vi "Update Settings.vi"(7 "Multicolumn Listbox Ref In":refnum<vi>, 8 "Error In":errorcluster, 11 "eHS Matrix Generation Session Ref In":refnum<data-value>) -> (0 "Error Out":errorcluster, 3 "eHS Matrix Generation Session Ref Out":refnum<data-value>)   [LabVIEW 2017]
uses:
  <vilib>/OPAL-RT/eHS Toolkit/eHS Matrix Generation/_Controls/eHS Core Index.ctl
  <vilib>/OPAL-RT/eHS Toolkit/eHS Matrix Generation/_Controls/eHS Matrix Generation Session.ctl
  <vilib>/OPAL-RT/eHS Toolkit/eHS Matrix Generation/_Controls/eHS Target Information.ctl
  <vilib>/OPAL-RT/eHS Toolkit/eHS Matrix Generation/_Controls/eHS Matrix Generation Parameters.ctl
  <vilib>/OPAL-RT/eHS Toolkit/eHS Matrix Generation/_Controls/eHS Circuit Analysis Data.ctl
  <vilib>/OPAL-RT/eHS Toolkit/eHS Matrix Generation/_Controls/eHS Core Settings.ctl
  <vilib>/OPAL-RT/eHS Toolkit/eHS Matrix Generation/_Controls/eHS Form Factor.ctl
  <vilib>/OPAL-RT/eHS Toolkit/eHS Matrix Generation/_Controls/eHS Model Information.ctl
  Update Settings States.ctl
  UI Refs.ctl
  ListBox/ListBox Action.ctl
  <vilib>/OPAL-RT/eHS Toolkit/eHS Matrix Generation/eHS Matrix Generation.lvlib
panel:
  out "Support Scenarios?":bool
  in  "Gs Settings":cluster{"SW#":i32, "Gs":sgl}[](array[cluster]) {"SW#" format="%02d"}
  in  "eHS Form Factor":T1=enum."eHSx64"
  out "Desired Ts (s)":string
  out "Cur eHS Form Factor":string
  out "eHS Core Index":string
  out "Model Name":string
  in  "Change Core":bool
  in  "Get Settings":bool
  in  "Update?":bool
  in  "Desired Gs":dbl
  out "Number of Switches":string
  in  "Same Gs for all Switches?":bool
  in  "Desired Ts (s)":dbl
  in  "Done":bool
  out "Minimum Achievable Ts (s)":string
  out "Display":string
  in  "Choose eHS Core Index":T2
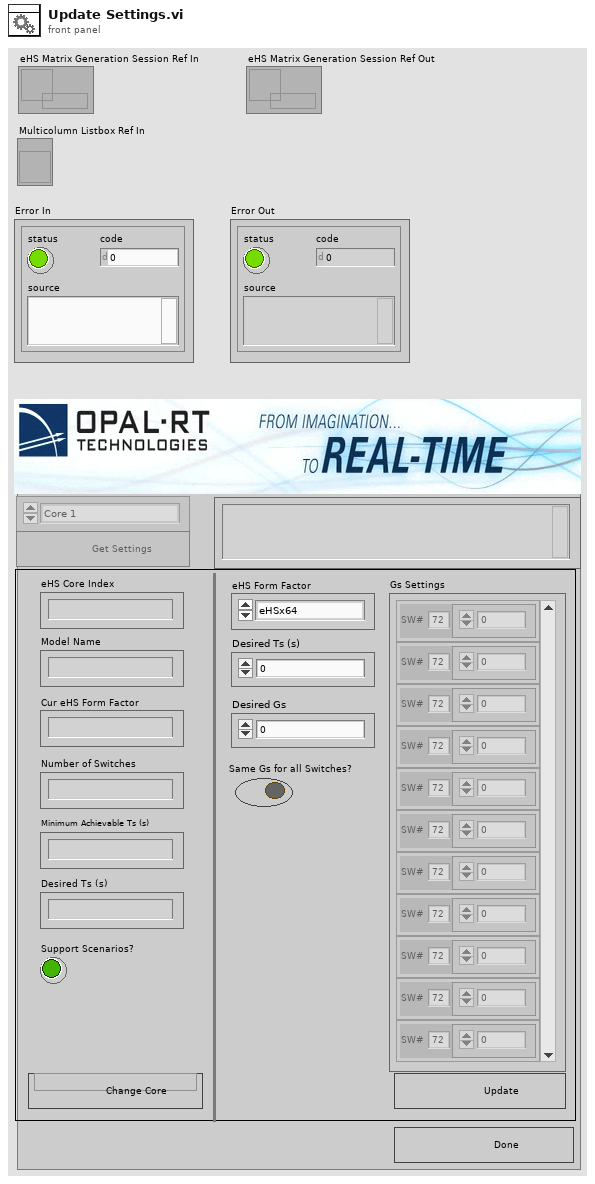
[diagram p1: front panel]
types:
  T1 = typedef "OPAL-RT eHS.lvlib/eHS Matrix Generation.lvlib/eHS Form Factor.ctl" = enum16{"eHSx16", "eHSx32", "eHSx64"}
  T2 = typedef "OPAL-RT eHS.lvlib/eHS Matrix Generation.lvlib/eHS Core Index.ctl" = enum16{"Core 1", "Core 2", "Core 3", "Core 4", "Core 5", "Core 6", "Core 7", "Core 8", "Core 9", "Core 10"}
  T3 = typedef "Update Settings States.ctl" = enum16{"Init", "Get Settings", "Update Settings", "Change Core", "Event Handler"}
  T4 = typedef "UI Refs.ctl" = cluster{"Choose Core":refnum<vi>, "Get Settings":refnum<vi>, "Change Core":refnum<vi>, "Form Factor":refnum<vi>, "Desired Ts":refnum<vi>, "Desired Gs":refnum<vi>, "Same Gs All":refnum<vi>, "Gs Settings":refnum<vi>, "Update":refnum<vi>}
  T5 = enum8{"Enabled", "Disabled", "Disabled and Grayed Out"}
  T6 = typedef "ListBox Action.ctl" = enum16{"Add", "Overwrite"}
  T7 = typedef "OPAL-RT eHS.lvlib/eHS Matrix Generation.lvlib/eHS Circuit Analysis Data.ctl" = cluster{"Number of Switches":string, "Desired Ts":string, "Gs":dbl[], "Min Ts":string}
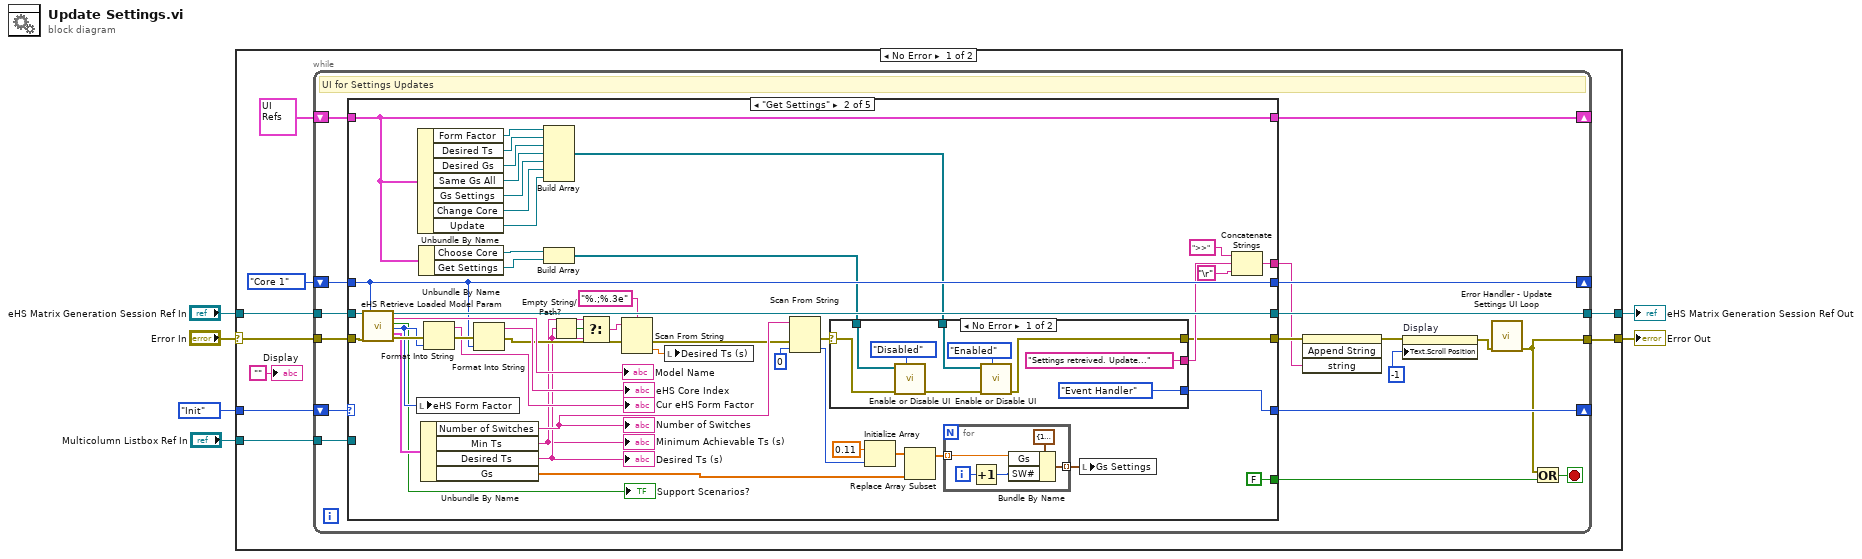
[diagram p0: block diagram]
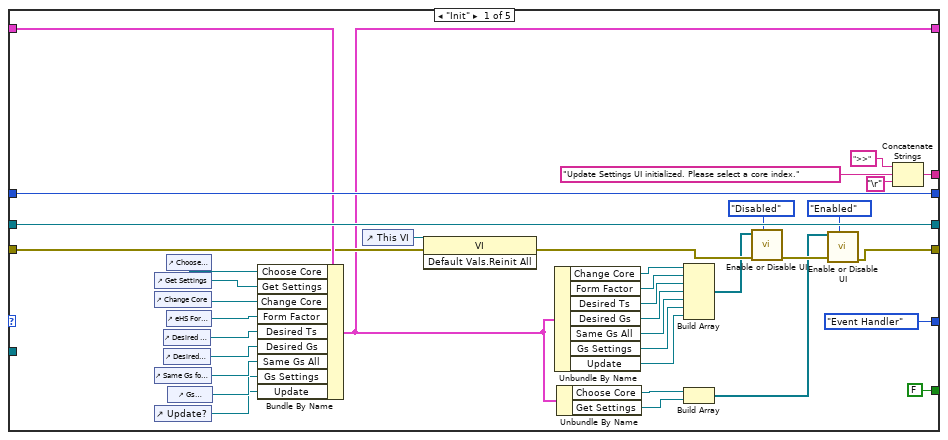
[diagram p2: hidden frame]
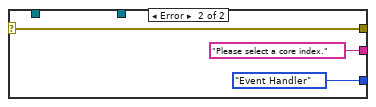
[diagram p3: hidden frame]
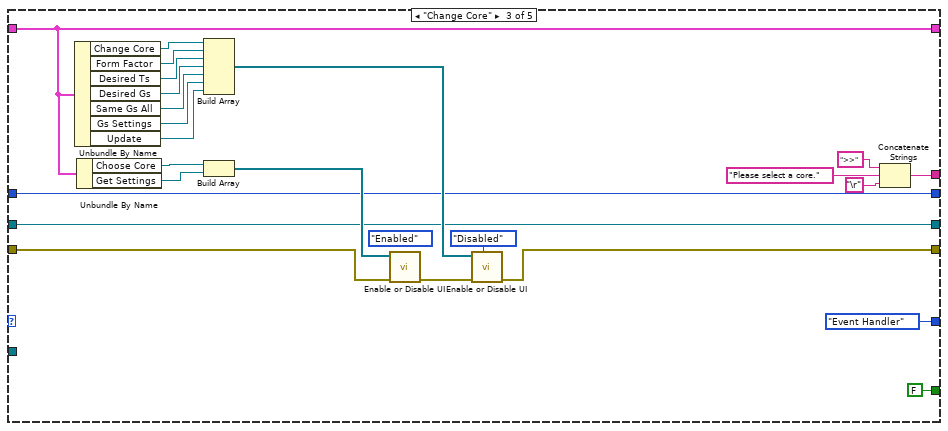
[diagram p4: hidden frame]
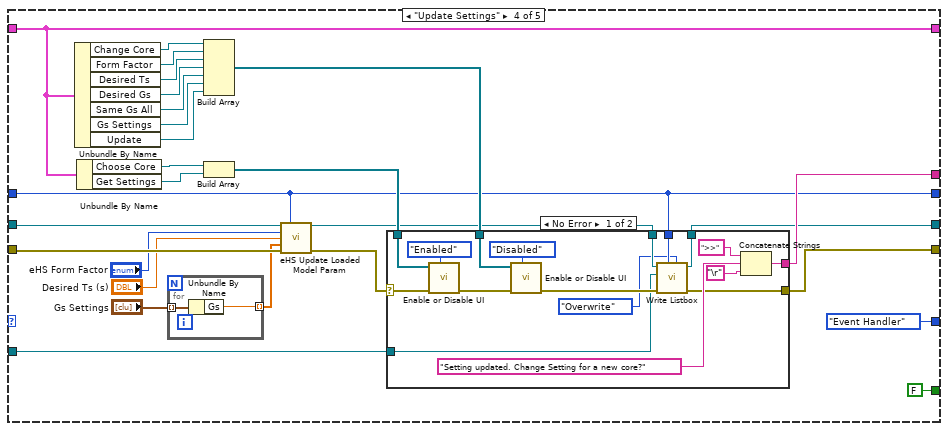
[diagram p5: hidden frame]
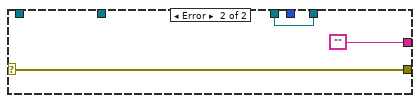
[diagram p6: hidden frame]
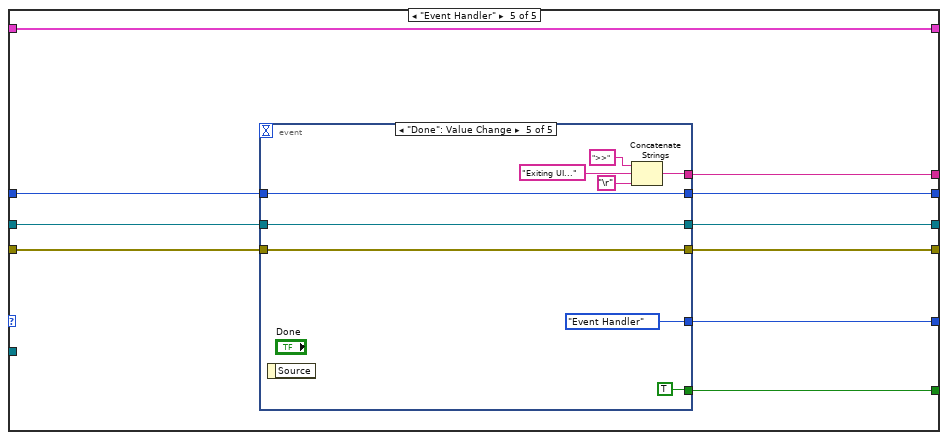
[diagram p7: hidden frame]
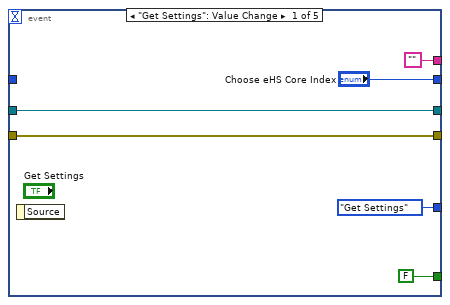
[diagram p8: hidden frame]
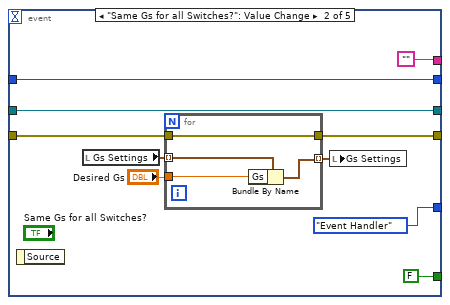
[diagram p9: hidden frame]
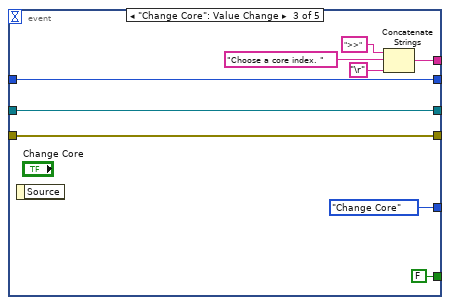
[diagram p10: hidden frame]
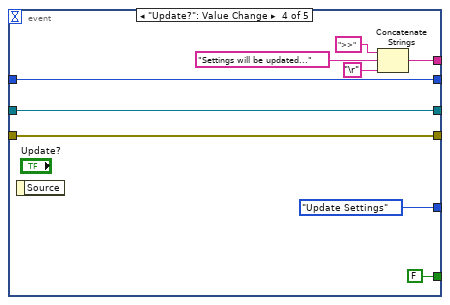
[diagram p11: hidden frame]
diagram:
  n1 = case shown="No Error" "Error In" {
    selector: "Error In" -> [w13 w267]
    tunnel: Update_Settings_States."Init" -> [w15 _]
    tunnel: "eHS Matrix Generation Session Ref In" -> [w14 w266]
    tunnel: [w9 w267] -> w3
    tunnel: [w11 w266] -> w2
    tunnel: "Multicolumn Listbox Ref In" -> [w7 _]
    frame No Error {
      n2 = while {
        tunnel: w14 -> [w32]
        tunnel: w13 -> [w31]
        shift-right: [w30] -> _
        shift-left: eHS_Core_Index."Core 1" ("eHS Core Index 2") -> [w29]
        shift-right: [w28] -> _
        shift-left: w15 -> [w33]
        tunnel: [w27] -> w11
        tunnel: [w16] -> w9
        shift-right: [w21] -> _
        shift-left: T4 {"Choose Core"=refnum, "Get Settings"=refnum, "Change Core"=refnum, "Form Factor"=refnum, "Desired Ts"=refnum, "Desired Gs"=refnum, "Same Gs All"=refnum, "Gs Settings"=refnum, "Update"=refnum} ("UI Refs") -> [w22]
        tunnel: w7 -> [w20]
        stop <- w18 stop-if-true
        # "UI for Settings Updates"
        n3 = case shown="\"Get Settings\"" w33 {
          tunnel: w32 -> [w69 w117 w143 w184 w214]
          tunnel: w31 -> [w52 w118 w145 w185 w212]
          tunnel: [w70 w110 w136 w161 w217] -> w30
          tunnel: w29 -> [w70 w110 w136 w161 w216]
          tunnel: [Update_Settings_States."Event Handler" w105 Update_Settings_States."Event Handler" Update_Settings_States."Event Handler" w218] -> w28
          tunnel: [w69 w116 w143 w162 w215] -> w27
          tunnel: [w65 w96 w139 w177 w211] -> w23
          tunnel: [w38 w93 w144 w178 w213] -> w26
          tunnel: [w35 w86 w148 w167 w209] -> w21
          tunnel: w22 -> [w63 w86 w148 w167 w209]
          tunnel: [FALSE FALSE FALSE FALSE w210] -> w17
          tunnel: w20 -> [_ _ _ w160 _]
          frame "Init" {
            n4 = control-ref of="Get Settings"() -> (w61:refnum<vi>)
            n5 = control-ref of="Change Core"() -> (w60:refnum<vi>)
            n6 = control-ref of="Same Gs for all Switches?"() -> (w56:refnum<vi>)
            n7 = control-ref of="Update?"() -> (w54:refnum<vi>)
            n8 = control-ref of="Desired Ts (s)"() -> (w58:refnum<vi>)
            n9 = control-ref of="Desired Gs"() -> (w57:refnum<vi>)
            n10 = control-ref of="Choose eHS Core Index"() -> (w62:refnum<vi>)
            n11 = control-ref of="eHS Form Factor"() -> (w59:refnum<vi>)
            n12 = control-ref of="Gs Settings"() -> (w55:refnum<vi>)
            n13 = Bundle By Name(cluster=w63, "Choose Core"=w62, "Get Settings"=w61, "Change Core"=w60, "Form Factor"=w59, "Desired Ts"=w58, "Desired Gs"=w57, "Same Gs All"=w56, "Gs Settings"=w55, "Update"=w54) -> (w35:T4)
            n14 = control-ref of="This VI"() -> (w53:refnum<vi>)
            n15 = invoke class="VI" method="Default Vals.Reinit All"(reference=w53, error in=w52) -> (error out=w39:errorcluster)  [unwired: 1 in, 2 out]
            n16 = Unbundle By Name(w35) -> ("Change Core"=w51:refnum<vi>, "Form Factor"=w50:refnum<vi>, "Desired Ts"=w49:refnum<vi>, "Desired Gs"=w48:refnum<vi>, "Same Gs All"=w47:refnum<vi>, "Gs Settings"=w46:refnum<vi>, "Update"=w45:refnum<vi>)
            n17 = Unbundle By Name(w35) -> ("Choose Core"=w41:refnum<vi>, "Get Settings"=w40:refnum<vi>)
            n18 = Build Array(w51, w50, w49, w48, w47, w46, w45) -> (w37:refnum<vi>[])
            n19 = Build Array(w41, w40) -> (w36:refnum<vi>[])
            n20 = call "Enable or Disable UI.vi"("Action"=T5."Disabled", "Error In"=w39, "Control Refs"=w37) -> ("Error Out"=w43:errorcluster)  [unwired: 8 in]
            n21 = call "Enable or Disable UI.vi"("Action"=T5."Enabled", "Error In"=w43, "Control Refs"=w36) -> ("Error Out"=w38:errorcluster)  [unwired: 8 in]
            n22 = Concatenate Strings(">>" ("string"), "Update Settings UI initialized. Please select a core index.", "\r") -> (w65:string)
          }
          frame "Get Settings" {
            n23 = call <vilib>:"eHS Retrieve Loaded Model Param.vi"("eHS Matrix Generation Session Ref In"=w117, "Error In"=w118, "eHS Core Index"=w110) -> ("eHS Matrix Generation Session Ref Out"=w116:refnum<data-value>, "Model Name"=→"Model Name":string, "Support Scenarios"=→"Support Scenarios?":bool, "eHS Form Factor"=w99:T1, "eHS Circuit Analysis Data"=w113:T7, "Error Out"=w114:errorcluster)  [unwired: 10 in, 1 out]
            n24 = local write "eHS Form Factor"(w99) -> ()
            n25 = Unbundle By Name(w86) -> ("Form Factor"=w92:refnum<vi>, "Desired Ts"=w91:refnum<vi>, "Desired Gs"=w90:refnum<vi>, "Same Gs All"=w89:refnum<vi>, "Gs Settings"=w88:refnum<vi>, "Change Core"=w85:refnum<vi>, "Update"=w78:refnum<vi>)
            n26 = Unbundle By Name(w86) -> ("Choose Core"=w84:refnum<vi>, "Get Settings"=w83:refnum<vi>)
            n27 = Unbundle By Name(w113) -> ("Number of Switches"=w108:string, "Min Ts"=w72:string, "Desired Ts"=w73:string, "Gs"=w101:dbl[])
            "Number of Switches" <- w108
            "Minimum Achievable Ts (s)" <- w72
            "Desired Ts (s)" <- w73
            n28 = Format Into String(error in=w114, w99) -> (resulting string=→"Cur eHS Form Factor":string, error out=w112:errorcluster)  [unwired: 2 in]
            n29 = Format Into String(error in=w112, w110) -> (resulting string=→"eHS Core Index":string, error out=w81:errorcluster)  [unwired: 2 in]
            n30 = Build Array(w92, w91, w90, w89, w88, w85, w78) -> (w87:refnum<vi>[])
            n31 = Build Array(w84, w83) -> (w82:refnum<vi>[])
            n32 = Empty String/Path?(string/path=w73) -> (empty?=w74:bool)
            n33 = Select(t=w72, s=w74, f=w73) -> (s? t:f=w75:string)
            n34 = Scan From String(format string="%.;%.3e", input string=w75, error in=w81) -> (error out=w80:errorcluster, output 1=w79:dbl)  [unwired: 2 in, 2 out]
            n35 = local write "Desired Ts (s)"(w79) -> ()
            n36 = Scan From String(input string=w108, error in=w80, default 1=0) -> (error out=w106:errorcluster, output 1=w104:i32)  [unwired: 2 in, 2 out]
            n37 = case shown="No Error" w106 {
              selector: w106 -> [w125 w128]
              tunnel: [Update_Settings_States."Event Handler" Update_Settings_States."Event Handler"] -> w105
              tunnel: ["Settings retreived. Update..." "Please select a core index."] -> w94
              tunnel: [w123 w128] -> w93
              tunnel: w87 -> [w120 _]
              tunnel: w82 -> [w119 _]
              frame No Error {
                n38 = call "Enable or Disable UI.vi"("Action"=T5."Disabled", "Error In"=w125, "Control Refs"=w119) -> ("Error Out"=w122:errorcluster)  [unwired: 8 in]
                n39 = call "Enable or Disable UI.vi"("Action"=T5."Enabled", "Error In"=w122, "Control Refs"=w120) -> ("Error Out"=w123:errorcluster)  [unwired: 8 in]
              }
              frame Error {
              }
            }
            n40 = Initialize Array(0.11, w104) -> (w102:dbl[])
            n41 = Replace Array Subset(array=w102, new element=w101) -> (w100:dbl[])  [unwired: 1 in]
            n42 = for {
              tunnel: [w134] -> w95 mode=indexing
              tunnel: w100 -> [w131] mode=indexing
              i -> [w135]
              n43 = Increment(x=w135) -> (x+1=w132:i32)
              n44 = Bundle By Name(cluster=cluster{"SW#":i32, "Gs":sgl} {"SW#"=1, "Gs"=0.11} ("Cluster"), "Gs"=w131, "SW#"=w132) -> (w134:cluster{"SW#":i32, "Gs":sgl})
            }
            n45 = local write "Gs Settings"(w95) -> ()
            n46 = Concatenate Strings(">>" ("string"), w94, "\r") -> (w96:string)
          }
          frame "Change Core" {
            (unwired) T5."Enabled" ("Action")
            n47 = Unbundle By Name(w148) -> ("Change Core"=w159:refnum<vi>, "Form Factor"=w158:refnum<vi>, "Desired Ts"=w157:refnum<vi>, "Desired Gs"=w156:refnum<vi>, "Same Gs All"=w155:refnum<vi>, "Gs Settings"=w154:refnum<vi>, "Update"=w153:refnum<vi>)
            n48 = Unbundle By Name(w148) -> ("Choose Core"=w152:refnum<vi>, "Get Settings"=w151:refnum<vi>)
            n49 = Build Array(w159, w158, w157, w156, w155, w154, w153) -> (w146:refnum<vi>[])
            n50 = Build Array(w152, w151) -> (w147:refnum<vi>[])
            n51 = call "Enable or Disable UI.vi"("Error In"=w145, "Control Refs"=w147) -> ("Error Out"=w149:errorcluster)  [unwired: 9 in]
            n52 = call "Enable or Disable UI.vi"("Action"=T5."Disabled", "Error In"=w149, "Control Refs"=w146) -> ("Error Out"=w144:errorcluster)  [unwired: 8 in]
            n53 = Concatenate Strings(">>" ("string"), "Please select a core." ("string"), "\r") -> (w139:string)
          }
          frame "Update Settings" {
            n54 = Unbundle By Name(w167) -> ("Change Core"=w176:refnum<vi>, "Form Factor"=w175:refnum<vi>, "Desired Ts"=w174:refnum<vi>, "Desired Gs"=w173:refnum<vi>, "Same Gs All"=w172:refnum<vi>, "Gs Settings"=w171:refnum<vi>, "Update"=w170:refnum<vi>)
            n55 = Unbundle By Name(w167) -> ("Choose Core"=w169:refnum<vi>, "Get Settings"=w168:refnum<vi>)
            n56 = for {
              tunnel: "Gs Settings" -> [w208] mode=indexing
              tunnel: [w207] -> w180 mode=indexing
              n57 = Unbundle By Name(w208) -> ("Gs"=w207:sgl)
            }
            n58 = Build Array(w176, w175, w174, w173, w172, w171, w170) -> (w165:refnum<vi>[])
            n59 = Build Array(w169, w168) -> (w166:refnum<vi>[])
            n60 = call <vilib>:"eHS Update Loaded Model Param.vi"("eHS Matrix Generation Session Ref In"=w184, "eHS Core Index"=w161, "eHS Form Factor"="eHS Form Factor", "Ts"="Desired Ts (s)", "Gs"=w180, "Error In"=w185) -> ("eHS Matrix Generation Session Ref Out"=w163:refnum<data-value>, "Error Out"=w179:errorcluster)  [unwired: 8 in]
            n61 = case shown="No Error" w179 {
              selector: w179 -> [w194 w206]
              tunnel: [w192 w206] -> w178
              tunnel: [w200 ""] -> w177
              tunnel: w166 -> [w196 _]
              tunnel: w165 -> [w195 _]
              tunnel: w163 -> [w191 w204]
              tunnel: [w190 w204] -> w162
              tunnel: w161 -> [w189 _]
              tunnel: w160 -> [w188 _]
              frame No Error {
                n62 = call "Enable or Disable UI.vi"("Action"=T5."Enabled", "Error In"=w194, "Control Refs"=w196) -> ("Error Out"=w198:errorcluster)  [unwired: 8 in]
                n63 = call "Enable or Disable UI.vi"("Action"=T5."Disabled", "Error In"=w198, "Control Refs"=w195) -> ("Error Out"=w193:errorcluster)  [unwired: 8 in]
                n64 = call "Write Listbox.vi"("Action"=ListBox_Action."Overwrite" ("ListBox Action"), "eHS Core Index"=w189, "Error In"=w193, "Multicolumn Listbox Ref In"=w188, "eHS Matrix Generation Session Ref In"=w191) -> ("Error Out"=w192:errorcluster, "eHS Matrix Generation Session Ref Out"=w190:refnum<data-value>)  [unwired: 4 in, 1 out]
                n65 = Concatenate Strings(">>" ("string"), "Setting updated. Change Setting for a new core?" ("string"), "\r") -> (w200:string)
              }
              frame Error {
              }
            }
          }
          frame "Event Handler" {
            n66 = event shown="[4] \"Done\": Value Change" {
              selector: _ -> [_ _ _ _ _]
              dyn-events: _ -> [_ _ _ _ _]
              timeout: _ -> [_ _ _ _ _]
              tunnel: [Update_Settings_States."Get Settings" Update_Settings_States."Event Handler" Update_Settings_States."Change Core" Update_Settings_States."Update Settings" Update_Settings_States."Event Handler"] -> w218
              tunnel: ["Choose eHS Core Index" w228 w240 w251 w265] -> w217
              tunnel: w216 -> [_ w228 w240 w251 w265]
              tunnel: [w222 w229 w242 w250 w259] -> w215
              tunnel: w214 -> [w222 w229 w242 w250 w259]
              tunnel: [w221 w230 w241 w249 w258] -> w213
              tunnel: w212 -> [w221 w231 w241 w249 w258]
              tunnel: ["" "" w244 w253 w262] -> w211
              tunnel: [FALSE FALSE FALSE FALSE TRUE] -> w210
              event "Get Settings": Value Change {
                n67 = event-data() -> ()  [unwired: 1 in, 1 out]
              }
              event "Same Gs for all Switches?": Value Change {
                n68 = event-data() -> ()  [unwired: 1 in, 1 out]
                n69 = local read "Gs Settings"() -> (w232:cluster{"SW#":i32, "Gs":sgl}[])
                n70 = for {
                  tunnel: w232 -> [w238] mode=indexing
                  tunnel: [w237] -> w234 mode=indexing
                  tunnel: "Desired Gs" -> [w236]
                  tunnel: w231 -> [w235]
                  tunnel: [w235] -> w230
                  n71 = Bundle By Name(cluster=w238, "Gs"=w236) -> (w237:cluster{"SW#":i32, "Gs":sgl})
                }
                n72 = local write "Gs Settings"(w234) -> ()
              }
              event "Change Core": Value Change {
                n73 = event-data() -> ()  [unwired: 1 in, 1 out]
                n74 = Concatenate Strings(">>" ("string"), "Choose a core index. ", "\r") -> (w244:string)
              }
              event "Update?": Value Change {
                n75 = event-data() -> ()  [unwired: 1 in, 1 out]
                n76 = Concatenate Strings(">>" ("string"), "Settings will be updated...", "\r") -> (w253:string)
              }
              event "Done": Value Change {
                n77 = event-data() -> ()  [unwired: 1 in, 1 out]
                n78 = Concatenate Strings(">>" ("string"), "Exiting UI...", "\r") -> (w262:string)
              }
            }
          }
        }
        n79 = invoke on="Display" class="Str" method="Append String"(error in=w26, "string"=w23) -> (error out=w25:errorcluster)  [unwired: 2 in, 3 out]
        n80 = property on="Display" class="Str"(error in=w25, "Text.Scroll Position"=-1) -> (error out=w19:errorcluster)  [unwired: 1 in, 1 out]
        n81 = call "Error Handler - Update Settings UI Loop.vi"("Error In"=w19) -> ("Error Out"=w16:errorcluster)  [unwired: 10 in]
        n82 = Or(x=w16, y=w17) -> (x .or. y?=w18:bool)
      }
      "Display" <- ""
    }
    frame Error {
    }
  }
  "eHS Matrix Generation Session Ref Out" <- w2
  "Error Out" <- w3
